vi "tcp test send.vi"() -> ()   [LabVIEW 2013]
panel:
  in  "停止按钮":bool
  in  "确定按钮":bool
  in  "Port":u16=6340 caption="PORT"
  in  "Machine":string="localhost" caption="IP"
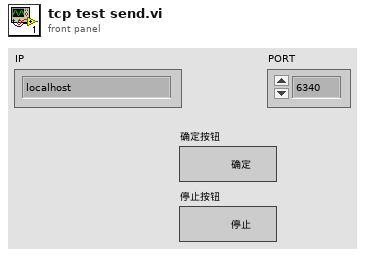
[diagram p1: front panel]
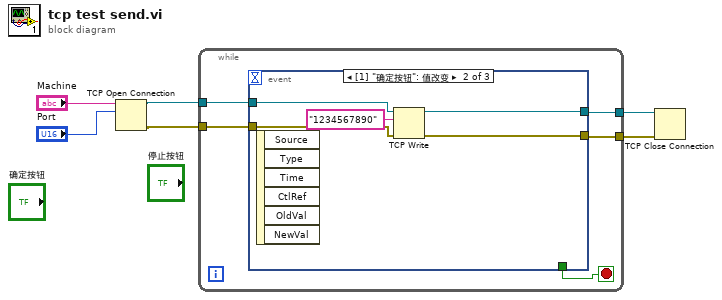
[diagram p0: block diagram]
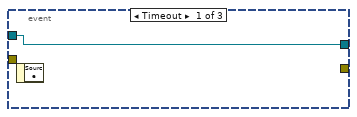
[diagram p2: hidden frame]
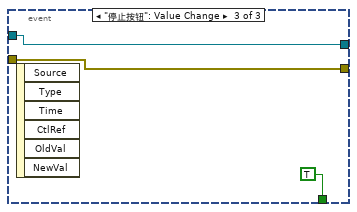
[diagram p3: hidden frame]
diagram:
  n1 = TCP Open Connection(address="Machine", remote port or service name="Port") -> (connection ID=w4:refnum<k5>, error out=w3:errorcluster)  [unwired: 3 in]
  n2 = while {
    tunnel: w4 -> [w11]
    tunnel: w3 -> [w10]
    tunnel: [w8] -> w2
    tunnel: [w7] -> w1
    stop <- w9 stop-if-true
    n3 = event shown="[1] \"确定按钮\": 值改变" {
      selector: _ -> [_ _ _]
      dyn-events: _ -> [_ _ _]
      timeout: _ -> [_ _ _]
      tunnel: w11 -> [w12 w17 w19]
      tunnel: w10 -> [_ w16 w18]
      tunnel: [_ w15 w18] -> w7
      tunnel: [w12 w14 w19] -> w8
      tunnel: [_ _ TRUE] -> w9
      event Timeout {
        n4 = event-data() -> ()  [unwired: 1 in, 1 out]
      }
      event "确定按钮": Value Change {
        n5 = event-data() -> ()  [unwired: 1 in, 6 out]
        n6 = TCP Write(connection ID=w17, data in="1234567890" ("数据输入"), error in (no error)=w16) -> (connection ID out=w14:refnum<k5>, error out=w15:errorcluster)  [unwired: 1 in, 1 out]
      }
      event "停止按钮": Value Change {
        n7 = event-data() -> ()  [unwired: 1 in, 6 out]
      }
    }
  }
  n8 = TCP Close Connection(connection ID=w2, error in (no error)=w1) -> ()  [unwired: 1 in, 2 out]
